vi "Tosca-Create Fade Out Matrix.vi"(0 "SignalManager in":refnum<class "SignalManager.lvclass">, 9 "npts":i32, 11 "error in (no error)":errorcluster) -> (4 "SignalManager out":refnum<class "SignalManager.lvclass">, 14 "fade out":dbl[][](array[numeric]), 15 "error out":errorcluster)   [LabVIEW 2020]
uses:
  epl-vi-lib/Signal Synthesis VIs/4th Generation/Classes/SignalManager/SignalManager.lvclass
  epl-vi-lib/Signal Synthesis VIs/4th Generation/Classes/SignalManager/SignalManager.lvclass/SignalManager.ctl
  epl-vi-lib/Signal Synthesis VIs/4th Generation/Classes/SignalManager/Read Channels.vi
  epl-vi-lib/Signal Synthesis VIs/4th Generation/Classes/SignalManager/Read Fs (Hz).vi
  epl-vi-lib/Signal Synthesis VIs/4th Generation/Classes/Channel/Channel.lvclass
  <vilib>/Analysis/NI_AALBase.lvlib
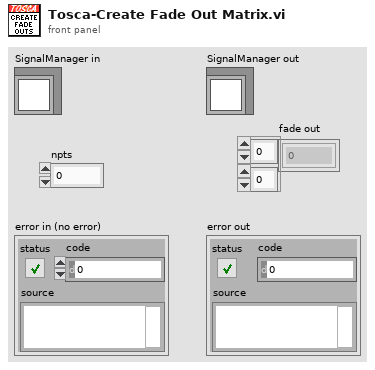
[diagram p1: front panel]
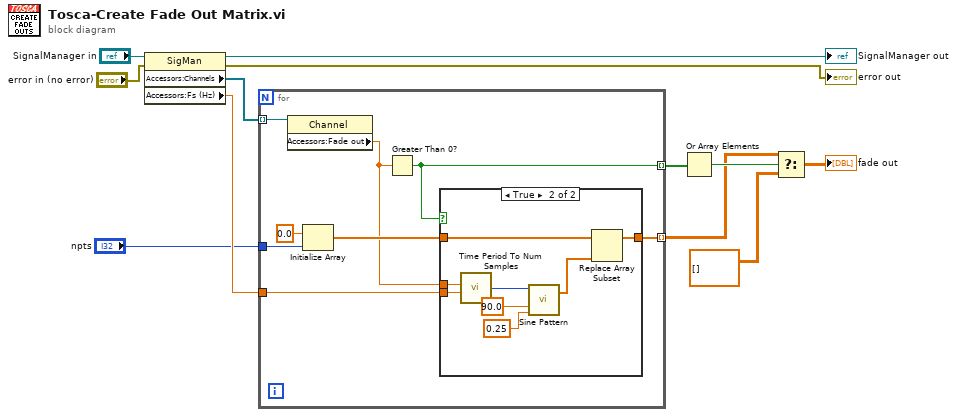
[diagram p0: block diagram]
diagram:
  n1 = property class="SigMan"(reference="SignalManager in", error in="error in (no error)") -> (reference out=→"SignalManager out":refnum<class "SignalManager.lvclass">, error out=→"error out":errorcluster, "Accessors:Channels"=w10:refnum<class "Channel.lvclass">[], "Accessors:Fs (Hz)"=w8:dbl)
  n2 = for {
    tunnel: w10 -> [w20] mode=indexing
    tunnel: [w13] -> w9 mode=indexing
    tunnel: w8 -> [w16]
    tunnel: "npts" -> [w15]
    tunnel: [w14] -> w3 mode=indexing
    n3 = property class="Channel"(reference=w20) -> ("Accessors:Fade out"=w17:dbl)  [unwired: 1 in, 2 out]
    n4 = Initialize Array(0.0 ("element"), w15) -> (w19:dbl[])
    n5 = Greater Than 0?(x=w17) -> (x > 0?=w13:bool)
    n6 = case shown="True" w13 {
      tunnel: w19 -> [w21 w26]
      tunnel: w17 -> [_ w24]
      tunnel: w16 -> [_ w23]
      tunnel: [w21 w22] -> w14
      frame False {
      }
      frame True {
        n7 = call "Time Period To Num Samples.vi"("Duration (ms)"=w24, "Sampling rate (Hz)"=w23) -> ("Samples"=w25:i32)  [unwired: 5 in]
        n8 = call <vilib>:"Sine Pattern.vi"("cycles"=0.25, "phase(degrees)"=90.0, "samples"=w25) -> ("Sinusoidal Pattern"=w28:dbl[])  [unwired: 1 in, 1 out]
        n9 = Replace Array Subset(array=w26, new element=w28) -> (w22:dbl[])  [unwired: 1 in]
      }
    }
  }
  n10 = Or Array Elements(Boolean array=w9) -> (logical OR=w4:bool)
  n11 = Select(t=w3, s=w4, f=dbl[][] []) -> (s? t:f=→"fade out":dbl[][])
